vi "Attributes to ID.vi"(1 "attributes":string) -> (0 "owner and ID":T1)   [LabVIEW 2017]
uses:
  Error Owner and ID.ctl
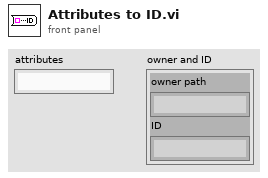
[diagram p1: front panel]
types:
  T1 = typedef "Error Owner and ID.ctl" = cluster{"owner path":string, "ID":string}
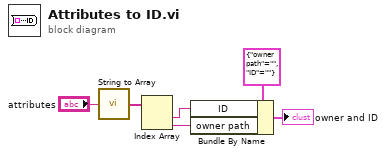
[diagram p0: block diagram]
diagram:
  n1 = call "String to Array.vi"("string"="attributes") -> ("array"=w6:string[])  [unwired: 1 in]
  n2 = Index Array(array=w6) -> (element #1=w5:string, element #2=w4:string)  [unwired: 2 in]
  n3 = Bundle By Name(cluster=T1 {"owner path"="", "ID"=""} ("owner errors"), "ID"=w5, "owner path"=w4) -> (→"owner and ID":T1)
